vi "Wait For Operation Complete.vi"(8 "error in (no error)":errorcluster, 10 "Maximum Time (5000ms)":u32=5000, 11 "VISA resource name":refnum<visa-resource-name>) -> (0 "error out":errorcluster, 3 "VISA resource name out":refnum<visa-resource-name>)   [LabVIEW 2013, in "Agilent 90000 Series.lvlib"]
doc: "Initiates a waveform acquisition. After you call this VI, the instrument leaves the Idle state and waits for a trigger.\n\n<B>Note:</B> Use this VI only with other low-level VIs. The high-level VIs automatically incorporate this functionality. This VI does not check the instrument status."
uses:
  Agilent 90000 Series.lvlib
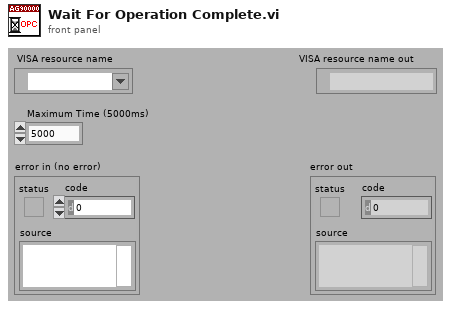
[diagram p1: front panel]
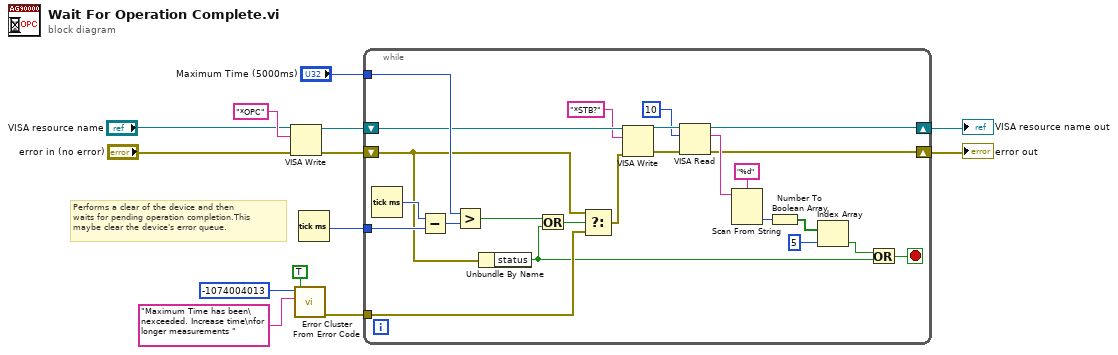
[diagram p0: block diagram]
diagram:
  # "Performs a clear of the device and then \nwaits for pending operation completion.This \nmaybe clear the device's error queue."
  n1 = VISA Write(VISA resource name="VISA resource name", write buffer="*OPC", error in (no error)="error in (no error)") -> (VISA resource name out=w5:refnum<visa-resource-name>, error out=w4:errorcluster)  [unwired: 1 out]
  n2 = call <vilib>:"Error Cluster From Error Code.vi"("show call chain? (False)"=TRUE, "error message (\"\")"="Maximum Time has been\nexceeded. Increase time\nfor longer measurements " ("error message (\"\")"), "error code (0)"=-1074004013) -> ("error out"=w9:errorcluster)  [unwired: 6 in]
  n3 = Tick Count (ms)() -> (millisecond timer value=w13:u32)
  n4 = while {
    tunnel: w13 -> [w36]
    tunnel: "Maximum Time (5000ms)" -> [w34]
    tunnel: w9 -> [w31]
    shift-right: [w23] -> w7
    shift-left: w5 -> [w29]
    shift-right: [w20] -> w6
    shift-left: w4 -> [w30]
    stop <- w19 stop-if-true
    n5 = Tick Count (ms)() -> (millisecond timer value=w37:u32)
    n6 = Subtract(x=w37, y=w36) -> (x-y=w35:u32)
    n7 = Greater?(x=w34, y=w35) -> (0:w33:bool)
    n8 = Unbundle By Name(w30) -> ("status"=w14:bool)
    n9 = Or(x=w33, y=w14) -> (x .or. y?=w32:bool)
    n10 = Select(t=w30, s=w32, f=w31) -> (s? t:f=w28:errorcluster)
    n11 = VISA Write(VISA resource name=w29, write buffer="*STB?", error in (no error)=w28) -> (VISA resource name out=w26:refnum<visa-resource-name>, error out=w25:errorcluster)  [unwired: 1 out]
    n12 = VISA Read(VISA resource name=w26, byte count=u32 10, error in (no error)=w25) -> (VISA resource name out=w23:refnum<visa-resource-name>, read buffer=w22:string, error out=w20:errorcluster)  [unwired: 1 out]
    n13 = Scan From String(format string="%d", input string=w22) -> (output 1=w18:i32)  [unwired: 3 in, 3 out]
    n14 = Number To Boolean Array(number=w18) -> (Boolean array=w17:bool[])
    n15 = Index Array(array=w17, index=5) -> (element=w15:bool)
    n16 = Or(x=w15, y=w14) -> (x .or. y?=w19:bool)
  }
  "error out" <- w6
  "VISA resource name out" <- w7
